vi "changeEXT.vi"(7 "Path":path, 10 "error in (no error)":errorcluster, 11 "New Extension":string) -> (2 "error out":errorcluster, 3 "Success?":bool, 5 "Out CSV Path":path)   [LabVIEW 2019]
uses:
  kernel32.dll
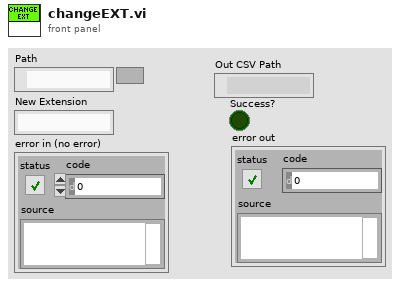
[diagram p1: front panel]
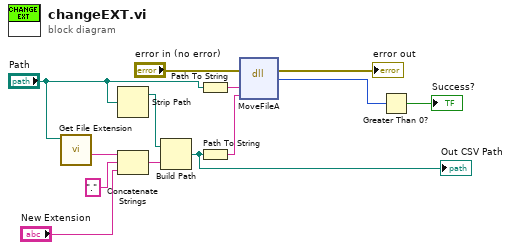
[diagram p0: block diagram]
diagram:
  n1 = call <vilib>:"Get File Extension.vi"("file"="Path") -> ("filename without extension"=w11:string)  [unwired: 6 in, 4 out]
  n2 = Strip Path(path="Path") -> (stripped path=w13:path)  [unwired: 1 out]
  n3 = Concatenate Strings(w11, ".", "New Extension") -> (w12:string)
  n4 = Build Path(base path=w13, name or relative path=w12) -> (appended path=w1:path)
  "Out CSV Path" <- w1
  n5 = Path To String(path="Path") -> (string=w10:string)
  n6 = Path To String(path=w1) -> (string=w9:string)
  n7 = dll-call lib="kernel32.dll" fn="MoveFileA"(error in="error in (no error)", "arg1"=w10, "arg2"=w9) -> (error out=→"error out":errorcluster, "return type"=w8:i32)  [unwired: 4 in, 1 out]
  n8 = Greater Than 0?(x=w8) -> (x > 0?=→"Success?":bool)
